vi "Build XY Plot Histogram (Core).vi"(4 "Bin Size":dbl, 5 "Align Histogram Bin":bool, 6 "Plot Index":i32, 7 "Max Number of Bins":i32, 8 "error in (no error)":errorcluster, 9 "Data Axis (Y: F)":bool, 10 "Mouse Click Coords":T1, 11 "XYGraph in":T2) -> (0 "error out":errorcluster, 1 "Message":string, 3 "Data Statistics":dbl[](array[numeric]))   [LabVIEW 2019, in "Histogram Window.lvlib"]
uses:
  Histogram Window.lvlib
  XY Graph Refnum.ctl
  <vilib>/Utility/miscctls.llb/LVPoint32TypeDef.ctl
  Plot Histogram.ctl
  Plot Style 3.ctl
  Histogram Window Q Element v2.ctl
  Histogram Window Q Action v2.ctl
  Data Statistics.ctl
  48084c95-8393-4bd0-bb26-e53c6117abf8.vi/9476f1cb-f14a-4b04-8e56-1278694a06a7.vi
  <vilib>/Analysis/NI_AALBase.lvlib
  <vilib>/Analysis/NI_AALPro.lvlib
  XY Graph Add-Ons.lvlib
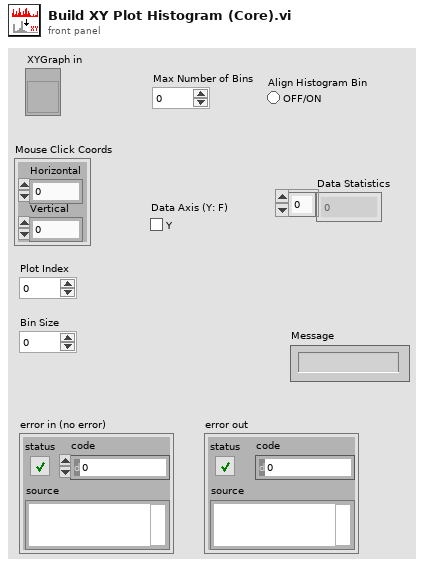
[diagram p1: front panel]
types:
  T1 = typedef "LVPoint32TypeDef.ctl" = cluster{"Horizontal":i32, "Vertical":i32}
  T2 = typedef "XY Graph Add-Ons.lvlib/XY Graph Refnum.ctl" = refnum<vi>
  T3 = typedef "Plot Style 3.ctl" = cluster{"Plot Style":enum16{"unchanged", "Line", "Symbol", "Line + Symbol", "Histogram", "Histogram + Symbol"}, "Histogram Type":enum16{"unchanged", "Left Bound", "Center", "Right Bound"}, "Line Tickness":enum16{"unchanged", "Thin", "1 pixel", "2 pixel", "3 pixel", "4 pixel", "5 pixel"}, "Line Style":enum16{"unchanged", "Plain", "Long Dash", "Short Dash", "Long-Short Dash", "Long-Short-Short Dash"}, "Point Style":enum16{"unchanged", "None", "Empty Circle", "Filled Circle", "Thick Circle", "Dotted Circle", "Empty Square", "Filled Square", "Thick Square", "Dotted Square", "Small Filled Square", "Dot", "Cross", "Tiny Cross", "Large X", "Small x", "Diamond", "Small Empty Square"}, "Line Color":u32, "Point Color":u32, "Anti-aliased":bool, "Line Color Chooser":enum16{"unchanged", "Color Box", "Color List"}, "Point Color Chooser":enum16{"unchanged", "Color Box", "Color List"}, "Line Color List":string, "Point Color List":string}
  T4 = typedef "Histogram Window.lvlib/Data Statistics.ctl" = cluster{"mean":dbl, "standard deviation":dbl, "variance":dbl, "rms value":dbl, "median":dbl, "mode":dbl, "max Value":dbl, "min Value":dbl, "# elements  ":dbl}
  T5 = typedef "Histogram Window.lvlib/Histogram Window Q Element v2.ctl" = cluster{"Histogram Window Q Action":T6, "Data":variant}
  T6 = typedef "Histogram Window.lvlib/Histogram Window Q Action v2.ctl" = enum16{"Initialization", "Add Histogram", "Delete Histogram", "Delete Selected Histograms", "Clear Graph", "Change Bin Size", "Invert Histogram", "Update Graph", "Edit Plot", "Plot Fit", "Export XYGraph to Notebook", "Select All Plots", "Deselect All Plots", "Invert Plots Selection", "Set Style of Selected Plots", "Save Plot", "Save Selected Plots", "Save All Plots", "Quit"}
  T7 = typedef "Histogram Window.lvlib/Plot Histogram.ctl" = cluster{"Plot Name":string, "Histogram":cluster{"Axis":dbl[], "Histogram":dbl[]}, "Plot Style":T3}
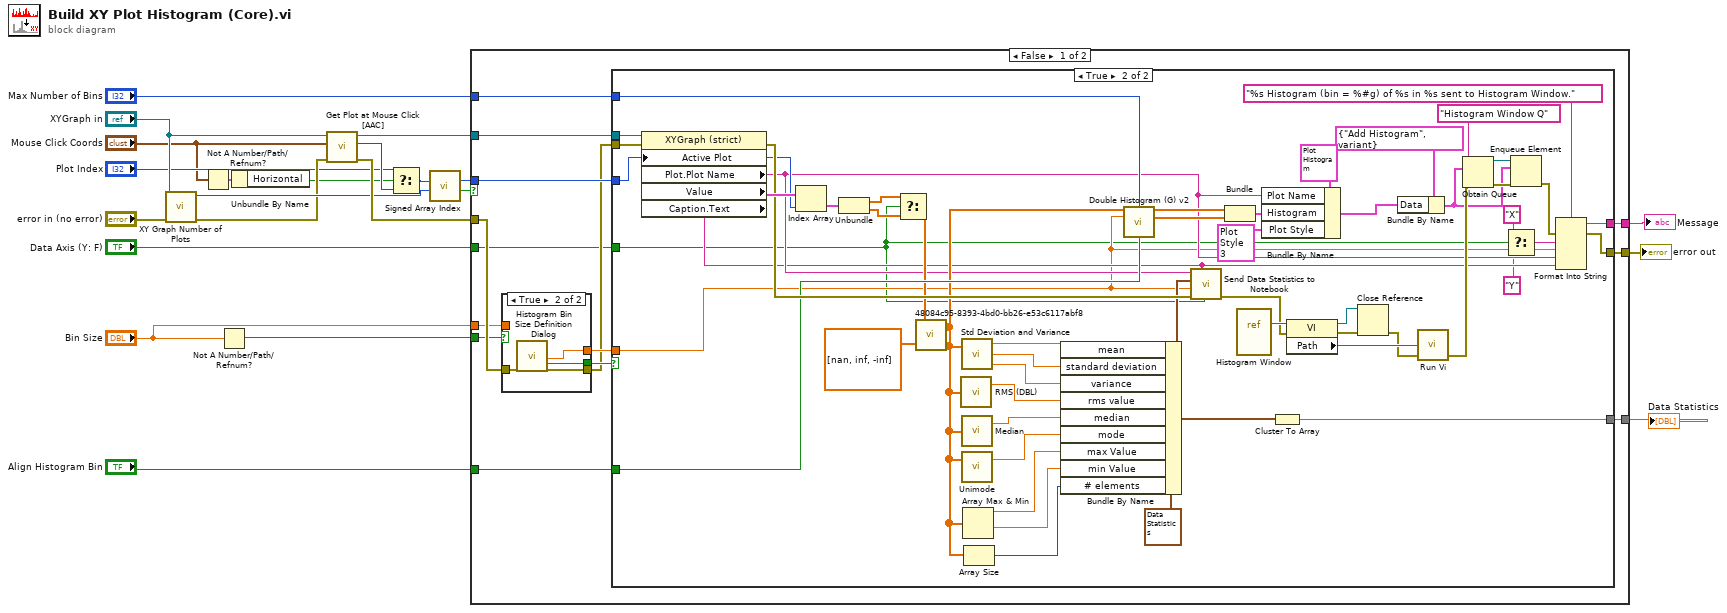
[diagram p0: block diagram]
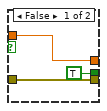
[diagram p3: hidden frame]
diagram:
  n1 = call "XY Graph Number of Plots.vi"("Error In"="error in (no error)", "XYGraph in"="XYGraph in") -> ("Error Out"=w14:errorcluster, "# Plots"=w17:i32)  [unwired: 8 in]
  n2 = Not A Number/Path/Refnum?(number/path/refnum="Mouse Click Coords") -> (NaN/Path/Refnum?=w6:cluster{"Horizontal":bool, "Vertical":bool})
  n3 = Not A Number/Path/Refnum?(number/path/refnum="Bin Size") -> (NaN/Path/Refnum?=w10:bool)
  n4 = Unbundle By Name(w6) -> ("Horizontal"=w7:bool)
  n5 = call "Get Plot at Mouse Click [AAC].vi"("error in (no error)"=w14, "Mouse Click Coordinates"="Mouse Click Coords", "XYGraph Ref"="XYGraph in") -> ("error out"=w19:errorcluster, "Plot at Coordinates"=w9:i32, "XYGraph Ref"=w3:T2)  [unwired: 2 in, 4 out]
  n6 = Select(t="Plot Index", s=w7, f=w9) -> (s? t:f=w15:i32)
  n7 = call "Signed Array Index.vi"("Array Size"=w17, "Array Index in"=w15) -> ("Out of Range?"=w18:bool, "Array Index out"=w16:i32)  [unwired: 8 in]
  n8 = case shown="False" w18 {
    tunnel: [w35 w99] -> w22
    tunnel: w3 -> [w36 _]
    tunnel: "Max Number of Bins" -> [w30 _]
    tunnel: w19 -> [w29 w99]
    tunnel: "Align Histogram Bin" -> [w28 _]
    tunnel: [w27 _] -> w4
    tunnel: w10 -> [w26 _]
    tunnel: "Bin Size" -> [w25 _]
    tunnel: w16 -> [w34 _]
    tunnel: "Data Axis (Y: F)" -> [w24 _]
    tunnel: [w23 _] -> w1
    frame False {
      n9 = case shown="True" w26 {
        tunnel: [w94 w98] -> w33
        tunnel: [TRUE ("OK") w97] -> w32
        tunnel: [w92 w96] -> w31
        tunnel: w29 -> [w92 w95]
        tunnel: w25 -> [w94 _]
        frame False {
        }
        frame True {
          n10 = call "Histogram Bin Size Definition Dialog.vi"("error in (no error)"=w95) -> ("Bin"=w98:dbl, "OK"=w97:bool, "error out"=w96:errorcluster)  [unwired: 16 in]
        }
      }
      n11 = case shown="True" w32 {
        tunnel: w36 -> [_ w91]
        tunnel: [w37 w52] -> w35
        tunnel: w34 -> [_ w66]
        tunnel: w33 -> [_ w47]
        tunnel: w31 -> [w37 w82]
        tunnel: w30 -> [_ w77]
        tunnel: w28 -> [_ w65]
        tunnel: [_ w59] -> w27
        tunnel: w24 -> [_ w44]
        tunnel: [_ w51] -> w23
        frame False {
        }
        frame True {
          n12 = property class="XYGraph (strict)"(reference=w91, error in=w82, "Active Plot"=w66) -> (error out=w79:errorcluster, "Plot.Plot Name"=w49:string, "Value"=w81:cluster{"X Array":dbl[], "Y Array":dbl[]}[], "Caption.Text"=w48:string)  [unwired: 1 out]
          n13 = Index Array(array=w81, index=w66) -> (element=w80:cluster{"X Array":dbl[], "Y Array":dbl[]})
          n14 = Unbundle(w80) -> ("X Array"=w56:dbl[], "Y Array"=w55:dbl[])
          n15 = Select(t=w56, s=w44, f=w55) -> (s? t:f=w54:dbl[])
          n16 = call "48084c95-8393-4bd0-bb26-e53c6117abf8.vi"("Element(s) to Remove"=dbl[] [nan, inf, -inf], "Input Array"=w54) -> ("Output Array"=w57:dbl[])  [unwired: 1 out]
          n17 = call <vilib>:"RMS (DBL).vi"("X"=w57) -> ("rms value"=w72:dbl)  [unwired: 1 out]
          n18 = call <vilib>:"Std Deviation and Variance.vi"("X"=w57) -> ("mean"=w75:dbl, "standard deviation"=w74:dbl, "variance"=w73:dbl)  [unwired: 1 in]
          n19 = call <vilib>:"Median.vi"("X"=w57) -> ("median"=w71:dbl)  [unwired: 1 out]
          n20 = call <vilib>:"Unimode.vi"("X"=w57) -> ("mode"=w70:dbl)  [unwired: 1 in, 1 out]
          n21 = Array Max & Min(array=w57) -> (max value=w69:dbl, min value=w68:dbl)  [unwired: 2 out]
          n22 = Array Size(array=w57) -> (size(s)=w67:i32)
          n23 = Bundle By Name(cluster=T4 {"mean"=0.0, "standard deviation"=0.0, "variance"=0.0, "rms value"=0.0, "median"=0.0, "mode"=0.0, "max Value"=0.0, "min Value"=0.0, "# elements  "=0.0} ("Data Statistics"), "mean"=w75, "standard deviation"=w74, "variance"=w73, "rms value"=w72, "median"=w71, "mode"=w70, "max Value"=w69, "min Value"=w68, "# elements"=w67) -> (w60:T4)
          n24 = call "Double Histogram (G) v2.vi"("Array"=w57, "Max Histogram Size (10^5)"=w77, "Bin Size (Sturge's Rule)"=w47, "Aligned Bins (F)"=w65) -> ("Axis"=w83:dbl[], "Histogram"=w84:dbl[])  [unwired: 9 in, 1 out]
          n25 = call "Send Data Statistics to Notebook.vi"("Data Axis (Y: F)"=w44, "Graph Caption"=w48, "Error In"=w79, "Bin"=w47, "Data Statistics"=w60, "Plot Name"=w49) -> ("Error Out"=w61:errorcluster)  [unwired: 5 in]
          n26 = Bundle("Axis"=w83, "Histogram"=w84) -> (w89:cluster{"Axis":dbl[], "Histogram":dbl[]})  [unwired: 1 in]
          n27 = vi-ref "Histogram Window.vi"() -> (w64:refnum<vi>)
          n28 = Bundle By Name(cluster=T7 {"Plot Name"="", "Histogram"={"Axis"=[], "Histogram"=[]}, "Plot Style"={"Plot Style"=enum."Histogram + Symbol", "Histogram Type"=enum."Right Bound", "Line Tickness"=enum."unchanged", "Line Style"=enum."unchanged", "Point Style"=enum."unchanged", "Line Color"=0, "Point Color"=0, "Anti-aliased"=FALSE, "Line Color Chooser"=enum."unchanged", "Point Color Chooser"=enum."unchanged", "Line Color List"="", "Point Color List"=""}} ("output cluster"), "Plot Name"=w49, "Histogram"=w89, "Plot Style"=T3 {"Plot Style"=enum."Histogram", "Histogram Type"=enum."Left Bound", "Line Tickness"=enum."1 pixel", "Line Style"=enum."Plain", "Point Style"=enum."None", "Line Color"=0, "Point Color"=0, "Anti-aliased"=TRUE, "Line Color Chooser"=enum."Color Box", "Point Color Chooser"=enum."unchanged", "Line Color List"="", "Point Color List"=""}) -> (w85:T7)
          n29 = Cluster To Array(cluster=w60) -> (array=w59:dbl[])
          n30 = property class="VI"(reference=w64, error in=w61) -> (reference out=w63:refnum<vi>, error out=w39:errorcluster, "Path"=w62:path)
          n31 = Close Reference(reference=w63, error in (no error)=w39) -> (error out=w38:errorcluster)
          n32 = Bundle By Name(cluster=T5 {"Histogram Window Q Action"=enum."Add Histogram", "Data"=variant} ("ALEX TT Histogram Q Element"), "Data"=w85) -> (w45:T5)
          n33 = call "Run Vi.vi"("VI Path"=w62, "error in (no error)"=w38) -> ("error out"=w78:errorcluster)  [unwired: 6 in, 1 out]
          n34 = Obtain Queue(name (unnamed)="Histogram Window Q", element data type=w45, error in (no error)=w78) -> (queue out=w88:refnum<queue>, error out=w86:errorcluster)  [unwired: 2 in, 1 out]
          n35 = Select(t="X" ("input 1"), s=w44, f="Y" ("input 1")) -> (s? t:f=w43:string)
          n36 = Enqueue Element(queue=w88, element=w45, error in (no error)=w86) -> (error out=w53:errorcluster)  [unwired: 1 in, 2 out]
          n37 = Format Into String(format string="%s Histogram (bin = %#g) of %s in %s sent to Histogram Window.", error in=w53, w43, w47, w49, w48) -> (resulting string=w51:string, error out=w52:errorcluster)  [unwired: 1 in]
        }
      }
    }
    frame True {
    }
  }
  "error out" <- w22
  "Data Statistics" <- w4
  "Message" <- w1
